vi "SavedSettingsSetTitleOrDescription.vi"(7 "Witch":u16(ring) items=["Title"=0, "Description"=3], 8 "error in (no error)":errorcluster, 9 "Value":string, 10 "Tag":string, 11 "TreeControl in":refnum<vi>) -> (0 "error out":errorcluster, 3 "reference out":refnum<vi>)   [LabVIEW 2021]
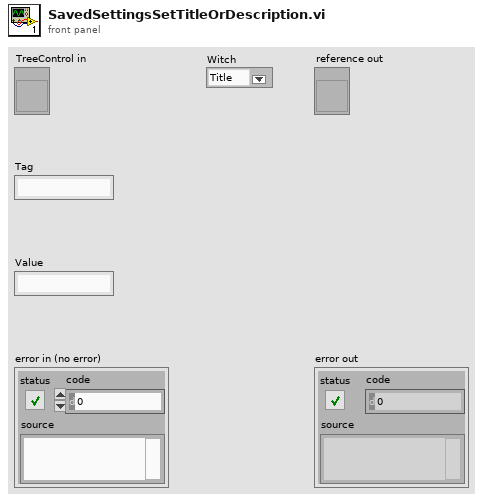
[diagram p1: front panel]
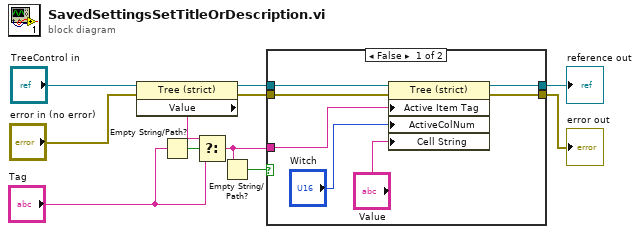
[diagram p0: block diagram]
diagram:
  n1 = property class="Tree (strict)"(reference="TreeControl in", error in="error in (no error)") -> (reference out=w10:refnum<vi>, error out=w9:errorcluster, "Value"=w5:string)
  n2 = Empty String/Path?(string/path="Tag") -> (empty?=w3:bool)
  n3 = Select(t=w5, s=w3, f="Tag") -> (s? t:f=w2:string)
  n4 = Empty String/Path?(string/path=w2) -> (empty?=w1:bool)
  n5 = case shown="False" w1 {
    tunnel: w10 -> [w17 w20]
    tunnel: w9 -> [w16 w19]
    tunnel: [w13 w19] -> w8
    tunnel: [w14 w20] -> w7
    tunnel: w2 -> [w15 _]
    frame False {
      n6 = property class="Tree (strict)"(reference=w17, error in=w16, "Active Item Tag"=w15, "ActiveColNum"="Witch", "Cell String"="Value") -> (reference out=w14:refnum<vi>, error out=w13:errorcluster)
    }
    frame True {
    }
  }
  "error out" <- w8
  "reference out" <- w7
